vi "SW_Log-transform_colors_array.vi"(2 "Image? (T)":bool, 3 "Log-transform? (F)":bool, 4 "Array or 24-bit pixmap in":u32[][](array[numeric])) -> (1 "Array or 24-bit pixmap out":u32[][](array[numeric]))   [LabVIEW 2018, in "Tracker.lvlib"]
uses:
  Tracker.lvlib
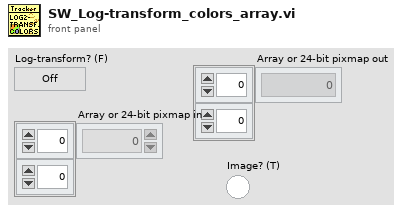
[diagram p1: front panel]
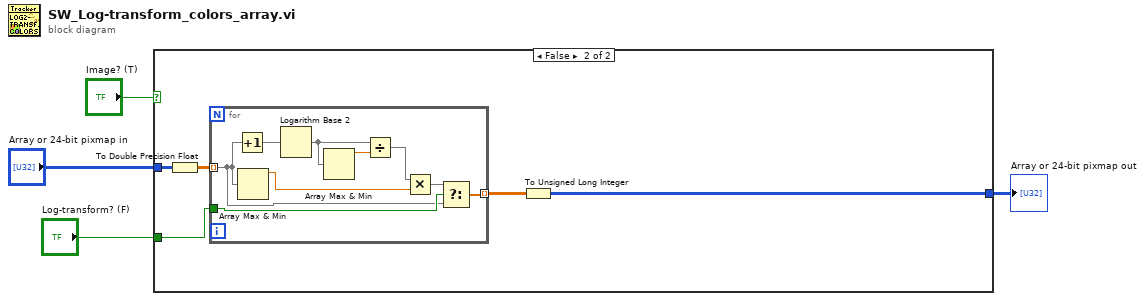
[diagram p0: block diagram]
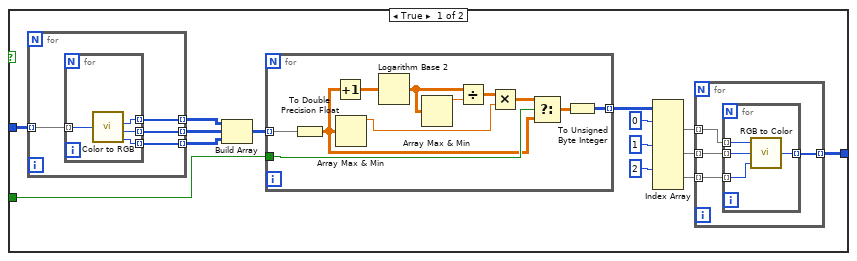
[diagram p2: hidden frame]
diagram:
  n1 = case shown="False" "Image? (T)" {
    tunnel: [w18 w46] -> w4
    tunnel: "Log-transform? (F)" -> [w17 w50]
    tunnel: "Array or 24-bit pixmap in" -> [w16 w49]
    frame True {
      n2 = for {
        tunnel: w16 -> [w22] mode=indexing
        tunnel: [w21] -> w5 mode=indexing
        tunnel: [w20] -> w6 mode=indexing
        tunnel: [w19] -> w7 mode=indexing
        n3 = for {
          tunnel: w22 -> [w26] mode=indexing
          tunnel: [w25] -> w21 mode=indexing
          tunnel: [w24] -> w20 mode=indexing
          tunnel: [w23] -> w19 mode=indexing
          n4 = call <vilib>:"Color to RGB.vi"("Color"=w26) -> ("R"=w25:u8, "G"=w24:u8, "B"=w23:u8)  [unwired: 1 out]
        }
      }
      n5 = Build Array(w5, w6, w7) -> (w8:u8[][][])
      n6 = for {
        tunnel: w8 -> [w45] mode=indexing
        tunnel: w17 -> [w43]
        tunnel: [w42] -> w9 mode=indexing
        n7 = To Double Precision Float(number=w45) -> (double precision float=w41:dbl[][])
        n8 = Increment(x=w41) -> (x+1=w35:dbl[][])
        n9 = Array Max & Min(array=w41) -> (max value=w37:dbl)  [unwired: 3 out]
        n10 = Logarithm Base 2(1:w35) -> (0:w40:dbl[][])
        n11 = Array Max & Min(array=w40) -> (max value=w39:dbl)  [unwired: 3 out]
        n12 = Divide(x=w40, y=w39) -> (x/y=w38:dbl[][])
        n13 = Multiply(x=w38, y=w37) -> (x*y=w36:dbl[][])
        n14 = Select(t=w36, s=w43, f=w41) -> (s? t:f=w44:dbl[][])
        n15 = To Unsigned Byte Integer(number=w44) -> (unsigned 8bit integer=w42:u8[][])
      }
      n16 = Index Array(array=w9, index (dim 0) #1=0 ("index (page)"), index (dim 0) #2=1 ("index (page)"), index (dim 0) #3=2 ("index (page)")) -> (element #1=w10:u8[][], element #2=w11:u8[][], element #3=w12:u8[][])  [unwired: 6 in]
      n17 = for {
        tunnel: w10 -> [w30] mode=indexing
        tunnel: w11 -> [w29] mode=indexing
        tunnel: w12 -> [w28] mode=indexing
        tunnel: [w27] -> w18 mode=indexing
        n18 = for {
          tunnel: w30 -> [w34] mode=indexing
          tunnel: w29 -> [w33] mode=indexing
          tunnel: w28 -> [w32] mode=indexing
          tunnel: [w31] -> w27 mode=indexing
          n19 = call <vilib>:"RGB to Color.vi"("B"=w32, "G"=w33, "R"=w34) -> ("Color"=w31:u32)
        }
      }
    }
    frame False {
      n20 = To Double Precision Float(number=w49) -> (double precision float=w48:dbl[][])
      n21 = for {
        tunnel: w50 -> [w59]
        tunnel: w48 -> [w52] mode=indexing
        tunnel: [w51] -> w47 mode=indexing
        n22 = Increment(x=w52) -> (x+1=w53:dbl[])
        n23 = Array Max & Min(array=w52) -> (max value=w55:dbl)  [unwired: 3 out]
        n24 = Logarithm Base 2(1:w53) -> (0:w58:dbl[])
        n25 = Array Max & Min(array=w58) -> (max value=w57:dbl)  [unwired: 3 out]
        n26 = Divide(x=w58, y=w57) -> (x/y=w56:dbl[])
        n27 = Multiply(x=w56, y=w55) -> (x*y=w54:dbl[])
        n28 = Select(t=w54, s=w59, f=w52) -> (s? t:f=w51:dbl[])
      }
      n29 = To Unsigned Long Integer(number=w47) -> (unsigned 32bit integer=w46:u32[][])
    }
  }
  "Array or 24-bit pixmap out" <- w4
